vi "Simulated Client.vi"(7 "Stop Signal":refnum<user-event>, 9 "period (ms)":i32=200, 10 "Client Name":string="Client1", 11 "project namespace":string="LabVIEWDemo") -> ()   [LabVIEW 2017]
uses:
  <vilib>/LabVIEW Open Source Project/MQTT Broker/Control Packets/CONNACK/Connect Return Code -- enum.ctl
  Car/Car State -- enum.ctl
  <vilib>/LabVIEW Open Source Project/MQTT Broker/Control Packets/CONNECT/ConnectFlags -- cluster.ctl
  Serializer.JKI-JSON/Serializer.JKI-JSON.lvclass
  C:/Program Files (x86)/National Instruments/LabVIEW 2017/vi.lib/LabVIEW Open Source Project/Serializer/Serializer/Serializer.lvclass
  WillPayload -- cluster.ctl
  <vilib>/LabVIEW Open Source Project/MQTT Broker/MQTT_Base/MQTT_Base.lvclass/MQTT_Base.ctl
  <vilib>/LabVIEW Open Source Project/MQTT Broker/Client/Client.lvclass/Client.ctl
  <vilib>/LabVIEW Open Source Project/MQTT Broker/Control Packets/ControlPacket/ControlPacket.lvclass/ControlPacket.ctl
  DisconnectPayload-- cluster.ctl
  e0c3b5cc-3527-4257-8471-923edf8b9748.vi
  <vilib>/LabVIEW Open Source Project/MQTT Broker/Control Packets/ControlPacket/Read Payload.vi
  <vilib>/LabVIEW Open Source Project/MQTT Broker/Client/Client.lvclass
  C:/Program Files (x86)/National Instruments/LabVIEW 2017/vi.lib/LabVIEW Open Source Project/MQTT Broker/MQTT_Base/MQTT_Base.lvclass
  <vilib>/LabVIEW Open Source Project/Serializer/Serializer.FlattenedString/Serializer.FlattenedString.lvclass
  <vilib>/LabVIEW Open Source Project/MQTT Broker/Control Packets/PUBLISH/PUBLISH.lvclass
  C:/Program Files (x86)/National Instruments/LabVIEW 2017/vi.lib/LabVIEW Open Source Project/MQTT Broker/Control Packets/ControlPacket/ControlPacket.lvclass
  <vilib>/LabVIEW Open Source Project/MQTT Broker/Control Packets/PUBLISH/getTopicName.vi
  <vilib>/LabVIEW Open Source Project/MQTT Broker/MQTT_Base/Decode Publish Package.vi
  <vilib>/LabVIEW Open Source Project/Serializer/Serializer/Serializer.lvclass
  <vilib>/LabVIEW Open Source Project/MQTT Broker/MQTT_Base/MQTT_Base.lvclass
  <vilib>/LabVIEW Open Source Project/MQTT Broker/Control Packets/CONNECT/CONNECT.lvclass
  <vilib>/addons/_JKI.lib/Serialization/JSON/JKI JSON Serialization.lvlib
  Car/Car.lvclass
  <vilib>/LabVIEW Open Source Project/MQTT Broker/Control Packets/CONNACK/CONNACK.lvclass
panel:
  in  "car state":T1
  out "error out":errorcluster
  in  "Force Close":bool
  in  "State History":i32(listbox)
  out "car state (get)":T1
  in  "subscribe":bool
  out "Topic":string
  out "Return Code":T2=enum."Server Unavailable"
  out "connected":bool
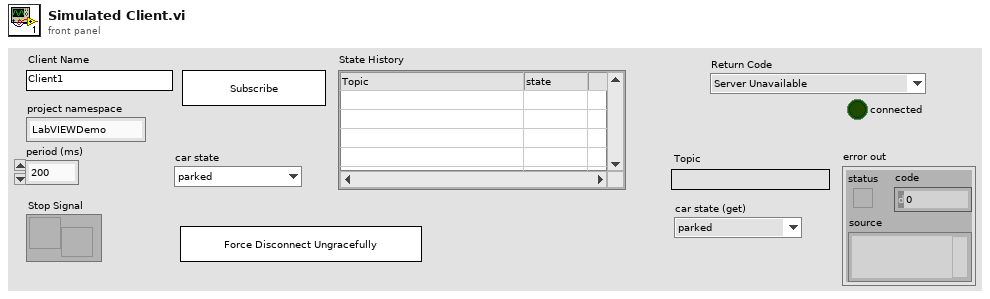
[diagram p1: front panel]
types:
  T1 = typedef "Car.lvclass/Car State -- enum.ctl" = enum16{"parked", "driving"}
  T2 = typedef "CONNACK.lvclass/Connect Return Code -- enum.ctl" = enum16{"Connection accepted", "Unacceptable protocol version", "Identifier Rejected", "Server Unavailable", "Bad Username or Password", "Not Authorized"}
  T3 = typedef "WillPayload -- cluster.ctl" = cluster{"message":string}
  T4 = typedef "CONNECT.lvclass/ConnectFlags -- cluster.ctl" = cluster{"Reserved":bool, "Clean Session":bool, "Will Flag":bool, "Will QoS 1":bool, "Will QoS 2":bool, "Will Retain":bool, "Password Flag":bool, "User Name Flag":bool}
  T5 = cluster{"Will Topic":string, "Will Message":string, "Username":string, "Password":string}
  T6 = typedef "MQTT Server.lvlib/Client.lvclass/Public Events -- cluster.ctl" = cluster{"Connection Status":refnum<user-event>, "Connected":refnum<user-event>, "Application Message":refnum<user-event>}
  T7 = typedef "DisconnectPayload-- cluster.ctl" = cluster{"timestamp":string}
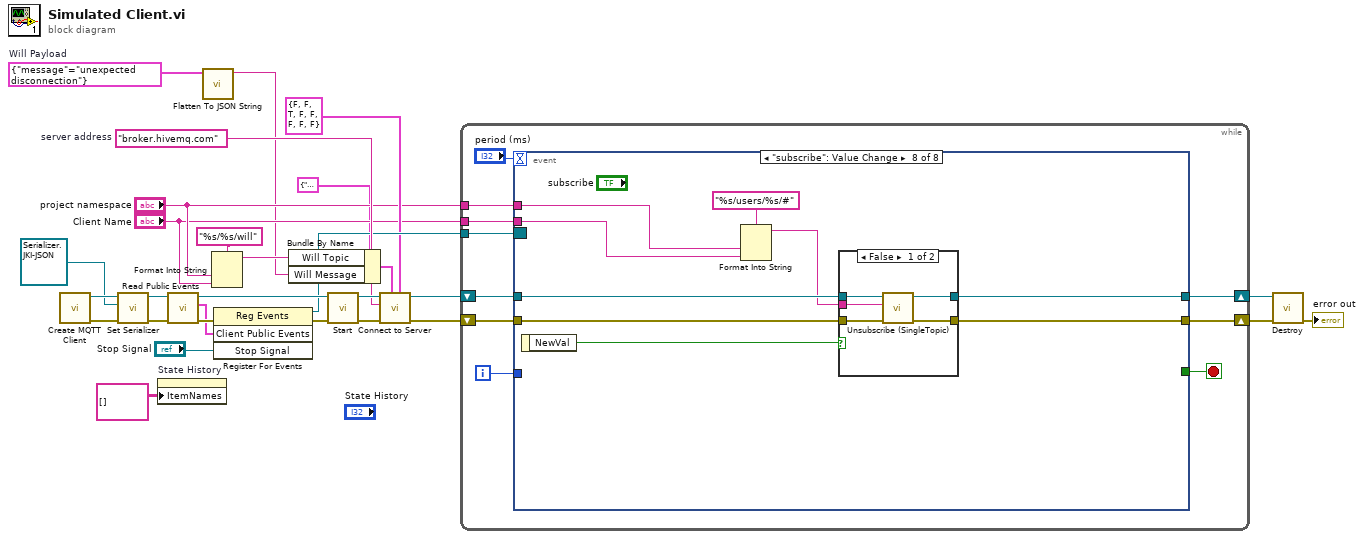
[diagram p0: block diagram]
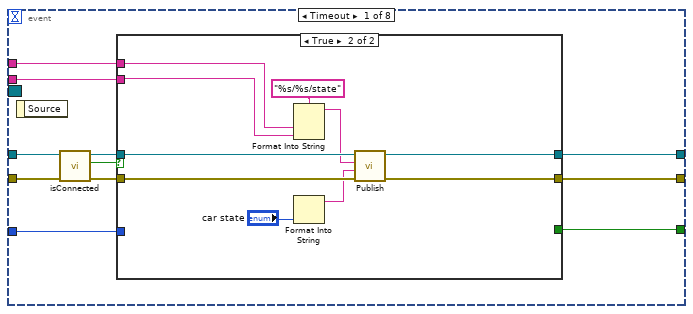
[diagram p2: hidden frame]
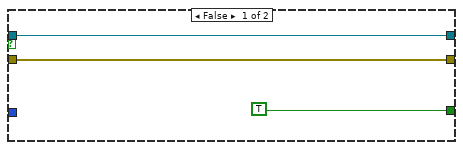
[diagram p3: hidden frame]
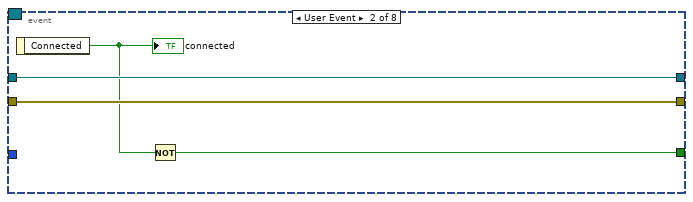
[diagram p4: hidden frame]
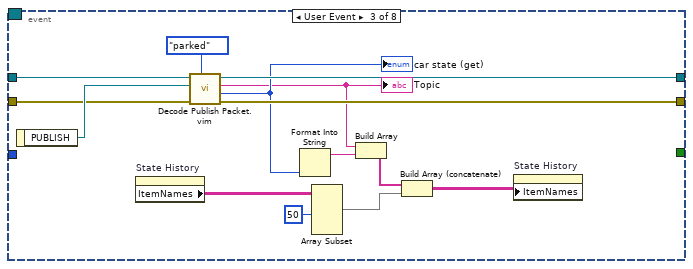
[diagram p5: hidden frame]
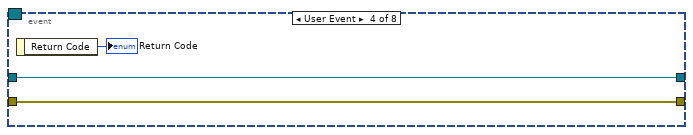
[diagram p6: hidden frame]
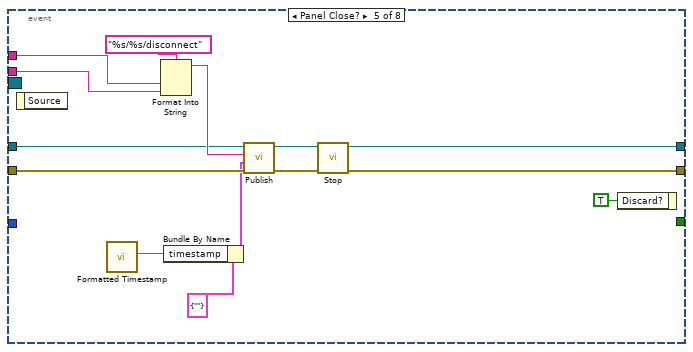
[diagram p7: hidden frame]
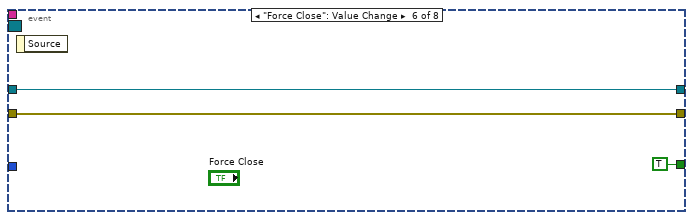
[diagram p8: hidden frame]
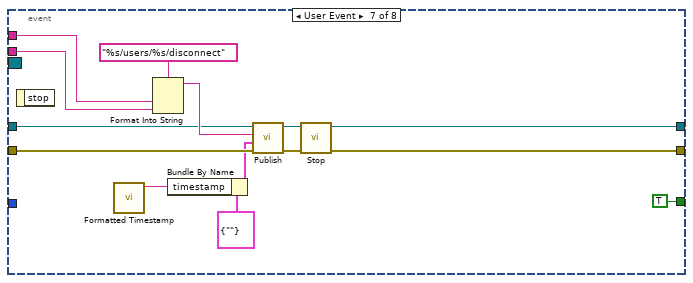
[diagram p9: hidden frame]
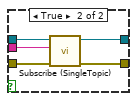
[diagram p10: hidden frame]
diagram:
  w2 = T3 {"message"="unexpected disconnection"}  # Will Payload
  w27 = "broker.hivemq.com"  # server address
  n1 = call <vilib>:"Create MQTT Client.vi"() -> ("error out"=w7:errorcluster, "Client out"=w5:refnum<class "Client.lvclass">)  [unwired: 10 in]
  n2 = call <vilib>:"Set Serializer.vi"("error in (no error)"=w7, "Serializer (default: Flattened String)"=refnum<class "Serializer.JKI-JSON.lvclass"> refnum ("Serializer.JKI-JSON.lvclass"), "MQTT_Base"=w5) -> ("error out"=w6:errorcluster, "MQTT_Base out"=w4:refnum<class "Client.lvclass">)  [unwired: 7 in]
  n3 = property on="State History" class="MCListbox (strict)"("ItemNames"=string[][] [] ("Item Names")) -> ()  [unwired: 2 in, 2 out]
  n4 = call <vilib>:"Read Public Events.vi"("error in (no error)"=w6, "Client in"=w4) -> ("error out"=w26:errorcluster, "Client Public Events"=w24:T6, "Client out"=w29:refnum<class "Client.lvclass">)  [unwired: 7 in]
  n5 = call <vilib>:"Flatten To JSON String.vi"("Variant"=w2) -> ("JSON String"=w1:string)  [unwired: 9 in, 1 out]
  n6 = Format Into String(format string="%s/%s/will", "project namespace", "Client Name") -> (resulting string=w13:string)  [unwired: 2 in, 1 out]
  n7 = register-events(error in=w26, w24, "Stop Signal") -> (reference out=w21:refnum<event-registration>, error out=w25:errorcluster)  [unwired: 1 in]
  n8 = Bundle By Name(cluster=T5 {"Will Topic"="", "Will Message"="", "Username"="", "Password"=""} ("Payload"), "Will Topic"=w13, "Will Message"=w1) -> (w11:T5)
  n9 = call <vilib>:"Start.vi"("error in (no error)"=w25, "MQTT_Base in"=w29) -> ("error out"=w23:errorcluster, "MQTT_Base out"=w28:refnum<class "Client.lvclass">)  [unwired: 7 in, 1 out]
  n10 = call <vilib>:"Connect to Server.vi"("Connect Flags"=T4 {"Reserved"=FALSE, "Clean Session"=FALSE, "Will Flag"=TRUE, "Will QoS 1"=FALSE, "Will QoS 2"=FALSE, "Will Retain"=FALSE, "Password Flag"=FALSE, "User Name Flag"=FALSE}, "Payload"=w11, "error in (no error)"=w23, "address (localhost)"=w27, "Client in"=w28) -> ("error out"=w20:errorcluster, "Client out"=w22:refnum<class "Client.lvclass">)  [unwired: 3 in, 2 out]
  n11 = while {
    shift-right: [w35] -> w10
    shift-left: w22 -> [w38]
    tunnel: w21 -> [w37]
    shift-right: [w34] -> w9
    shift-left: w20 -> [w36]
    tunnel: "project namespace" -> [w32]
    tunnel: "Client Name" -> [w30]
    i -> [w31]
    stop <- w33 stop-if-true
    n12 = event shown="[7] \"subscribe\": Value Change" {
      selector: w37 -> [_ _ _ _ _ _ _ _]
      dyn-events: _ -> [_ _ _ _ _ _ _ _]
      timeout: "period (ms)" -> [_ _ _ _ _ _ _ _]
      tunnel: w38 -> [w50 w67 w81 w83 w93 w101 w108 w124]
      tunnel: w36 -> [w49 w66 w78 w82 w91 w100 w106 w122]
      tunnel: [w47 w67 w80 w83 w97 w101 w113 w123] -> w35
      tunnel: [w45 w66 w77 w82 w96 w100 w114 w121] -> w34
      tunnel: [w41 w64 _ _ _ TRUE TRUE _] -> w33
      tunnel: w32 -> [w44 _ _ _ w89 _ w110 w120]
      tunnel: w31 -> [w43 _ _ _ _ _ _ _]
      tunnel: w30 -> [w40 _ _ _ w88 _ w109 w116]
      event Timeout {
        n13 = event-data() -> ()  [unwired: 1 in, 1 out]
        n14 = call <vilib>:"isConnected.vi"("error in (no error)"=w49, "Client in"=w50) -> ("error out"=w46:errorcluster, "connected"=w42:bool, "Client out"=w48:refnum<class "Client.lvclass">)  [unwired: 7 in]
        n15 = case shown="True" w42 {
          tunnel: w48 -> [w53 w63]
          tunnel: [w53 w62] -> w47
          tunnel: w46 -> [w52 w61]
          tunnel: [w52 w60] -> w45
          tunnel: w44 -> [_ w58]
          tunnel: w43 -> [_ _]
          tunnel: [TRUE _] -> w41
          tunnel: w40 -> [_ w56]
          frame False {
          }
          frame True {
            n16 = Format Into String(format string="%s/%s/state", w58, w56) -> (resulting string=w57:string)  [unwired: 2 in, 1 out]
            n17 = Format Into String("car state") -> (resulting string=w55:string)  [unwired: 3 in, 1 out]
            n18 = call <vilib>:"Publish.vi"("error in (no error)"=w61, "Payload"=w55, "Topic Name (empty: Payload name)"=w57, "Client in"=w63) -> ("error out"=w60:errorcluster, "Client out"=w62:refnum<class "Client.lvclass">)  [unwired: 5 in, 1 out]
          }
        }
      }
      event User Event {
        n19 = event-data() -> ("Connected"=w65:bool)  [unwired: 1 in]
        "connected" <- w65
        n20 = Not(x=w65) -> (.not. x?=w64:bool)
      }
      event User Event {
        n21 = event-data() -> ("PUBLISH"=w79:refnum<class "PUBLISH.lvclass">)  [unwired: 1 in]
        n22 = property on="State History" class="MCListbox (strict)"() -> ("ItemNames"=w71:string[][])  [unwired: 2 in, 2 out]
        n23 = call "Decode Publish Packet.vim"("Payload type"=Car_State_--_enum."parked" ("car state"), "error in (no error)"=w78, "PUBLISH"=w79, "Client in"=w81) -> ("error out"=w77:errorcluster, "Payload"=w76:T1, "Topic"=w75:string, "Client out"=w80:refnum<class "Client.lvclass">)  [unwired: 4 in]
        "Topic" <- w75
        "car state (get)" <- w76
        n24 = Format Into String(w76) -> (resulting string=w74:string)  [unwired: 3 in, 1 out]
        n25 = Array Subset(array=w71, length (row)=50 ("length")) -> (w70:string[][])  [unwired: 3 in]
        n26 = Build Array(w75, w74) -> (w73:string[])
        n27 = Build Array (concatenate)(w73, w70) -> (w72:string[][])
        n28 = property on="State History" class="MCListbox (strict)"("ItemNames"=w72) -> ()  [unwired: 2 in, 2 out]
      }
      event User Event {
        n29 = event-data() -> ("Return Code"=→"Return Code":T2)  [unwired: 1 in]
      }
      event Panel Close? {
        n30 = event-data() -> ()  [unwired: 1 in, 1 out]
        n31 = call "Formatted Timestamp.vi"() -> ("String Formatted timestamp"=w86:string)  [unwired: 11 in]
        n32 = Format Into String(format string="%s/%s/disconnect", w89, w88) -> (resulting string=w94:string)  [unwired: 2 in, 1 out]
        n33 = Bundle By Name(cluster=T7 {"timestamp"=""} ("Disconnect payload"), "timestamp"=w86) -> (w85:T7)
        n34 = call <vilib>:"Publish.vi"("error in (no error)"=w91, "Payload"=w85, "Topic Name (empty: Payload name)"=w94, "Client in"=w93) -> ("error out"=w90:errorcluster, "Client out"=w92:refnum<class "Client.lvclass">)  [unwired: 5 in, 1 out]
        n35 = call <vilib>:"Stop.vi"("error in (no error)"=w90, "MQTT_Base in"=w92) -> ("error out"=w96:errorcluster, "MQTT_Base out"=w97:refnum<class "Client.lvclass">)  [unwired: 7 in, 1 out]
        n36 = event-data("Discard?"=TRUE) -> ()  [unwired: 1 in, 1 out]
      }
      event "Force Close": Value Change {
        n37 = event-data() -> ()  [unwired: 1 in, 1 out]
      }
      event User Event {
        n38 = event-data() -> ()  [unwired: 1 in, 1 out]
        n39 = call "Formatted Timestamp.vi"() -> ("String Formatted timestamp"=w102:string)  [unwired: 11 in]
        n40 = Format Into String(format string="%s/users/%s/disconnect", w110, w109) -> (resulting string=w111:string)  [unwired: 2 in, 1 out]
        n41 = Bundle By Name(cluster=T7 {"timestamp"=""} ("Disconnect payload"), "timestamp"=w102) -> (w103:T7)
        n42 = call <vilib>:"Publish.vi"("error in (no error)"=w106, "Payload"=w103, "Topic Name (empty: Payload name)"=w111, "Client in"=w108) -> ("error out"=w105:errorcluster, "Client out"=w107:refnum<class "Client.lvclass">)  [unwired: 5 in, 1 out]
        n43 = call <vilib>:"Stop.vi"("error in (no error)"=w105, "MQTT_Base in"=w107) -> ("error out"=w114:errorcluster, "MQTT_Base out"=w113:refnum<class "Client.lvclass">)  [unwired: 7 in, 1 out]
      }
      event "subscribe": Value Change {
        n44 = event-data() -> ("NewVal"=w117:bool)  [unwired: 1 in]
        n45 = Format Into String(format string="%s/users/%s/#", w120, w116) -> (resulting string=w118:string)  [unwired: 2 in, 1 out]
        n46 = case shown="False" w117 {
          tunnel: w124 -> [w129 w134]
          tunnel: [w127 w133] -> w123
          tunnel: w122 -> [w126 w132]
          tunnel: [w125 w131] -> w121
          tunnel: w118 -> [w128 w130]
          frame False {
            n47 = call <vilib>:"Unsubscribe (SingleTopic).vi"("error in (no error)"=w126, "Topic Filter"=w128, "MQTT_Base in"=w129) -> ("error out"=w125:errorcluster, "MQTT_Base out"=w127:refnum<class "Client.lvclass">)  [unwired: 7 in]
          }
          frame True {
            n48 = call <vilib>:"Subscribe (SingleTopic).vi"("error in (no error)"=w132, "Topic Filter"=w130, "MQTT_Base in"=w134) -> ("error out"=w131:errorcluster, "MQTT_Base out"=w133:refnum<class "Client.lvclass">)  [unwired: 7 in]
          }
        }
      }
    }
  }
  n49 = call-dynamic "Destroy.vi"("error in (no error)"=w9, "MQTT_Base in"=w10) -> ("error out"=→"error out":errorcluster)  [unwired: 8 in, 1 out]
